vi "Get Color .NET.vi"(11 "Color in":refnum<class "Color.lvclass">) -> (2 "Color .NET":refnum<k24>, 3 "Color out":refnum<class "Color.lvclass">)   [LabVIEW 2024, in "Color.lvclass"]
uses:
  Color.lvclass
  Color.lvclass/Color.ctl
  System.Drawing
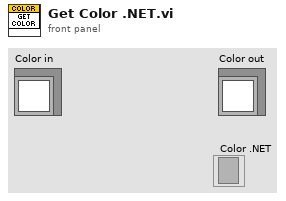
[diagram p1: front panel]
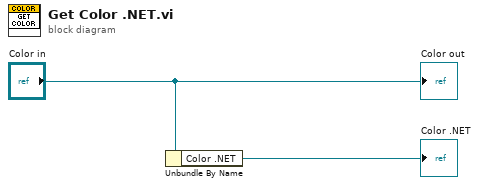
[diagram p0: block diagram]
diagram:
  n1 = Unbundle By Name("Color in") -> ("Color .NET"=→"Color .NET":refnum<k24>)
  "Color out" <- "Color in"
